vi "Calculate moves.vi"(7 "Position":refnum<class "Position.lvclass">, 8 "error in (no error)":errorcluster, 10 "Source":T1={"File"=enum."d", "Rank"=enum."4"}, 11 "Pawn in":refnum<class "Pawn.lvclass">) -> (0 "error out":errorcluster, 2 "Moves":refnum<class "Move.lvclass">[](array[class]), 3 "Pawn out":refnum<class "Pawn.lvclass">)   [LabVIEW 2016, in "Chesslib.lvlib" / "Pawn.lvclass"]
uses:
  Pawn.lvclass
  Moves/Move/Move.lvclass
  typedef/Square.ctl
  typedef/File.ctl
  typedef/Rank.ctl
  Position/Position.lvclass
  Chesslib.lvlib
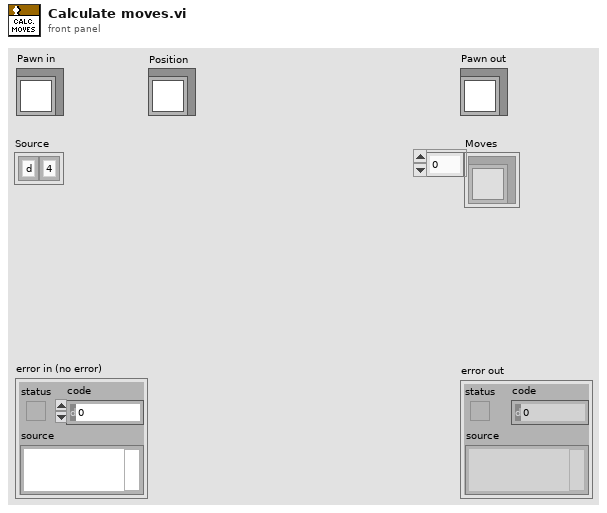
[diagram p1: front panel]
types:
  T1 = typedef "Chesslib.lvlib/Square.ctl" = cluster{"File":T2, "Rank":T3}
  T2 = typedef "Chesslib.lvlib/File.ctl" = enum8{"a", "b", "c", "d", "e", "f", "g", "h"}
  T3 = typedef "Chesslib.lvlib/Rank.ctl" = enum8{"1", "2", "3", "4", "5", "6", "7", "8"}
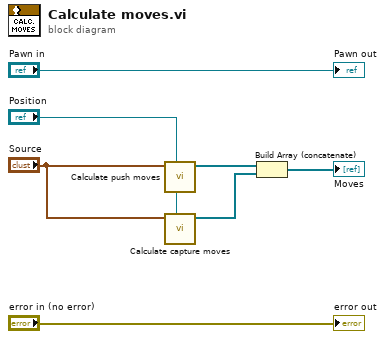
[diagram p0: block diagram]
diagram:
  n1 = call "Calculate push moves.vi"("Position in"="Position", "Source"="Source") -> ("Push moves"=w6:refnum<class "Move.lvclass">[])  [unwired: 9 in]
  n2 = call "Calculate capture moves.vi"("Position in"="Position", "Source"="Source") -> ("Capture moves"=w3:refnum<class "Move.lvclass">[])  [unwired: 9 in]
  n3 = Build Array (concatenate)(w6, w3) -> (→"Moves":refnum<class "Move.lvclass">[])
  "error out" <- "error in (no error)"
  "Pawn out" <- "Pawn in"
